vi "LVClass_Image get image data Uxx.vi"(0 "Image in":refnum<class "Image.lvclass">, 11 "error in (no error)":errorcluster) -> (4 "Image out":refnum<class "Image.lvclass">, 6 "Image data out":u32[][](array[numeric]), 15 "error out":errorcluster)   [LabVIEW 2020, in "Image.lvclass"]
doc: "Get pixels buffer from 32-bit Image.\n\n--------------------------------------------------------------------------------\n\n<B>ImageIn </B> : Image object.\n<B>ImageOut </B> : Image object.\n<B>buffer </B> : Pixel buffer.\n<B>ErrorIn </B> : Error\n<B>ErrorOut </B> : Error\n\n--------------------------------------------------------------------------------"
uses:
  Image.lvclass
  Point2D.ctl
  Image.lvclass/Image.ctl
  LVClass_Image Read Image.vi
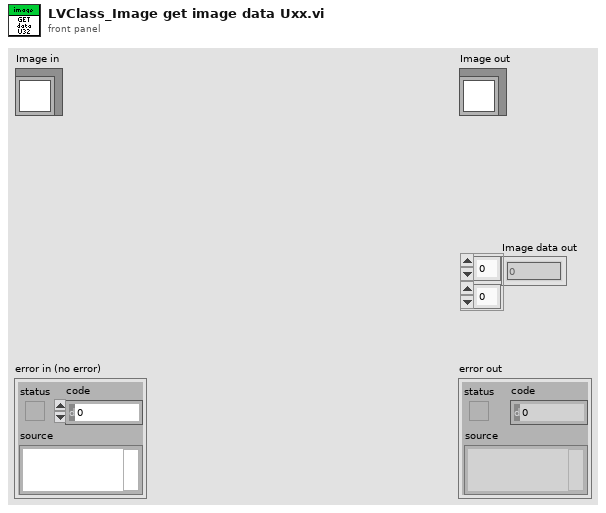
[diagram p1: front panel]
types:
  T1 = typedef "Point2D.ctl" = cluster{"X":u32, "Y":u32}
  T2 = typedef "Struct_Image.ctl" = cluster{"Image_Handler":T3, "Number of bits":T4, "ImageSize":T1}
  T3 = typedef "ClassID.ctl" = i64
  T4 = typedef "Data alignment enum.ctl" = enum16{"8", "16", "32"}
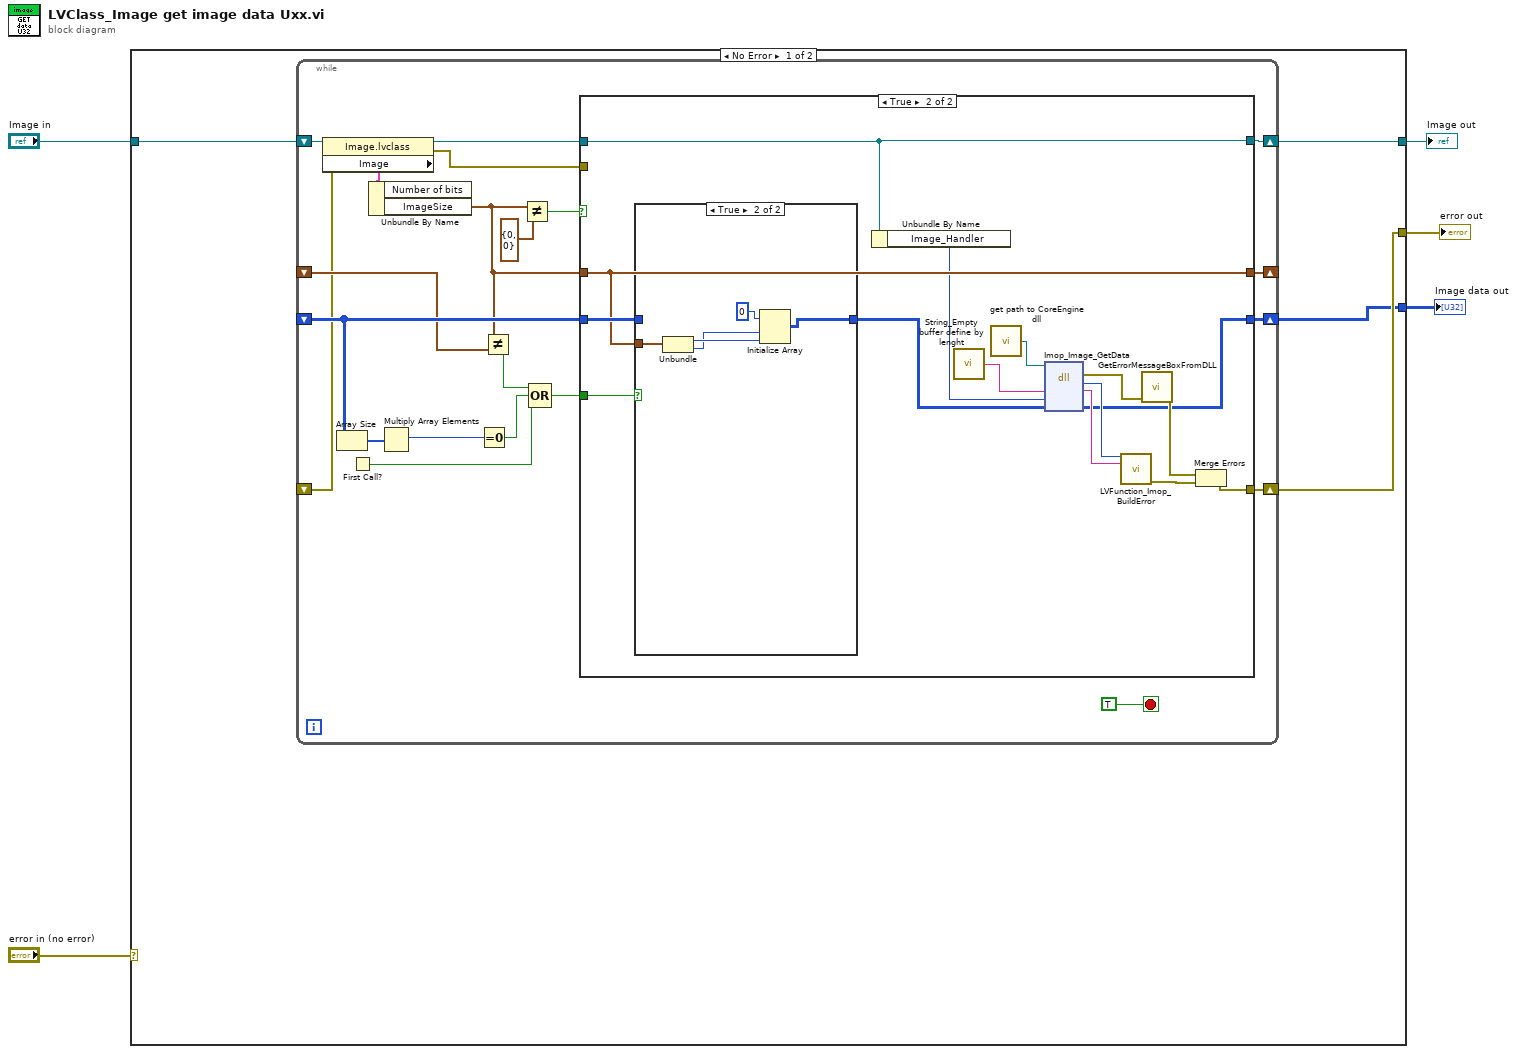
[diagram p0: block diagram]
diagram:
  n1 = case shown="No Error" "error in (no error)" {
    selector: "error in (no error)" -> [_ w57]
    tunnel: [w8 w57] -> w4
    tunnel: [w7 w56] -> w2
    tunnel: "Image in" -> [w9 w56]
    tunnel: [w6 _] -> w1
    frame No Error {
      n2 = while {
        shift-right: [w30] -> w6
        shift-left: _ -> [w28]
        shift-right: [w22] -> w7
        shift-left: w9 -> [w18]
        shift-right: [w21] -> w8
        shift-left: _ -> [w17]
        shift-right: [w14] -> _
        shift-left: _ -> [w20]
        stop <- TRUE stop-if-true
        n3 = property class="Image.lvclass"(reference=w18, error in=w17) -> (reference out=w19:refnum<class "Image.lvclass">, error out=w12:errorcluster, "Image"=w13:T2)
        n4 = Array Size(array=w28) -> (size(s)=w27:i32[])
        n5 = First Call?() -> (First Call?: T/F=w24:bool)
        n6 = Unbundle By Name(w13) -> ("ImageSize"=w11:T1)  [unwired: 1 out]
        n7 = Multiply Array Elements(1:w27) -> (0:w26:i32)
        n8 = Equal To 0?(x=w26) -> (x = 0?=w25:bool)
        n9 = Not Equal?(x=w11, y=w20) -> (x != y?=w10:bool)
        n10 = Not Equal?(x=w11, y=T1 {"X"=0, "Y"=0}) -> (x != y?=w15:bool)
        n11 = Compound Arithmetic op=OR(w10, w25, w24) -> (w23:bool)
        n12 = case shown="True" w15 {
          tunnel: [w34 w35] -> w30
          tunnel: w28 -> [w34 w49]
          tunnel: w23 -> [_ w48]
          tunnel: [w33 w47] -> w22
          tunnel: [w32 w46] -> w21
          tunnel: w19 -> [w33 w47]
          tunnel: w12 -> [w32 _]
          tunnel: w11 -> [w31 w45]
          tunnel: [w31 w45] -> w14
          frame False {
          }
          frame True {
            n13 = case shown="True" w48 {
              tunnel: [w50 w55] -> w36
              tunnel: w49 -> [w50 _]
              tunnel: w45 -> [_ w54]
              frame False {
              }
              frame True {
                n14 = Unbundle(w54) -> ("X"=w53:u32, "Y"=w52:u32)
                n15 = Initialize Array(u32 0 ("element"), w52, w53) -> (w55:u32[][])
              }
            }
            n16 = Unbundle By Name(w47) -> ("Image_Handler"=w44:T3)
            n17 = call "String_Empty buffer define by lenght.vi"() -> ("Empty buffer"=w37:string)  [unwired: 1 in]
            n18 = call "get path to CoreEngine dll.vi"() -> ("path to c_interface_vc100.dll"=w38:path)  [unwired: 12 in, 3 out]
            n19 = dll-call lib="D:/soft/HASO_v3/SVN_trunk/ImOpCoreEngine4_LV2011/DLLs/c_interface_vc100.dll" fn="Imop_Image_GetData"(path in=w38, "message"=w37, "Image compat"=w44, "Image data"=w36) -> (error out=w39:errorcluster, "return type"=w41:i32, "message"=w40:string, "Image data"=w35:u32[][])  [unwired: 3 in, 1 out]
            n20 = call "LVFunction_Imop_BuildError.vi"("code"=w41, "String to Prepend to source (\"\")"=w40) -> ("error out"=w43:errorcluster)  [unwired: 13 in]
            n21 = call "GetErrorMessageBoxFromDLL.vi"("error IN"=w39) -> ("error OUT"=w42:errorcluster)  [unwired: 10 in]
            n22 = Merge Errors(w42, w43) -> (w46:errorcluster)
          }
        }
      }
    }
    frame Error {
    }
  }
  "error out" <- w4
  "Image out" <- w2
  "Image data out" <- w1
